vi "AVARVAREI.vi"() -> ()   [LabVIEW 2025]
panel:
  in  "stop":bool
  out "H 4":string
  in  "V 4":bool[](array[boolean])
  out "H2":string
  in  "V 2":bool[](array[boolean])
  out "H 3":string
  in  "V 3":bool[](array[boolean])
  out "H 1":string
  in  "V 1":bool[](array[boolean])
  # "SISTEM DE CONVERSIE DIN BINAR IN HEHAZECIMAL"
  # "CITIREA CODULUI BINAR DE JOS IN SUS/DE LA DREAPTA LA STANGA"
  # "Algoritm de conversie din binar in zecimal\n1 0  0 0 0 1 0 0 (Binar) =132 (Zecimal) = 84 (hexazecimal)\n7 6 5 4 3 2 1 0 - pozitii in sistemul de conversie binar-zecimal\n7 6 5 4 3 2 1 0 - pozitii in vector/ array labVieW\n\n1*2^7+ 0*2^6+.....+ 1*2^2+...0*2^0=132\nMultiply, Add, Power of Two, Subtract\n\nFor loop-parcurgerea elementelor din vector\nN= nr maxim de iteratii=nr elemente vector\n\nIndex Tunnel=inlocuieste utilizarea a 2 functii:\n-index array=permite extragerea elementelor din vector\n-array size\n\nContor i(for loop)=0,1,2,3,4,5,6,7\n\nPower of Two\n-input: contor i\n-output: 2^0, 2^1, 2^2,....\n\nAlgoritm de conversie din zecimal in hexazecimal\n-->apelam functie din LavVIEW - Number to Hexazecimal\n\nShift Registers\n-->acceseaza elementele din iteratiile anterioare(for loop)\n\nBoolean to(0,1)--> conversie T/F la 1/0"
  # "CITIREA CODULUI BINAR DE SUS IN JOS/DE LA STANGA SPRE DREAPTA"
  # "Algoritm de conversie din binar in zecimal\n0 0 1 0 0 0 0 1 (Binar) = 33 (Zecimal) = 21 (hexazecimal)\n7 6 5 4 3 2 1 0 - pozitii in sistemul de conversie binar-zecimal\n0 1 2 3 4 5 6 7- pozitii in vector/ array labVieW\n\nPower of Two\n-input: contor N-1-I\ni=0-->n=8-->n-1-i=8-1-0=7\ni=1-->n=8-->n-1-i=8-1-1=6\n-output: 2^7, 2^6, 2^5....\n\nAlgoritm de conversie din zecimal in hexazecimal\n-->apelam functie din LavVIEW - Number to Hexazecimal"
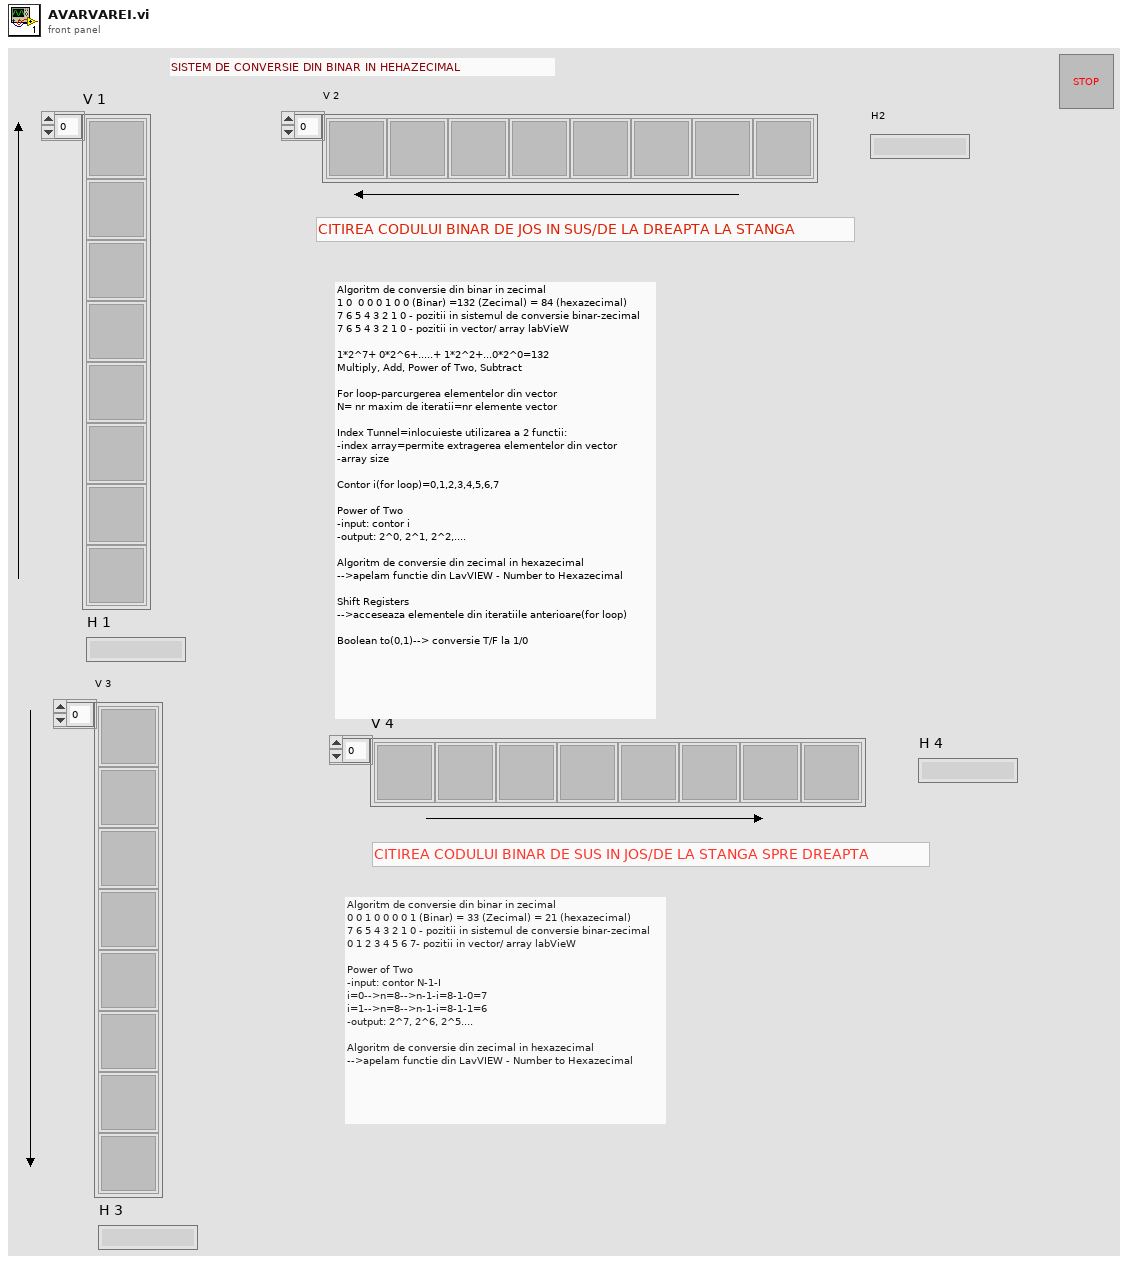
[diagram p1: front panel]
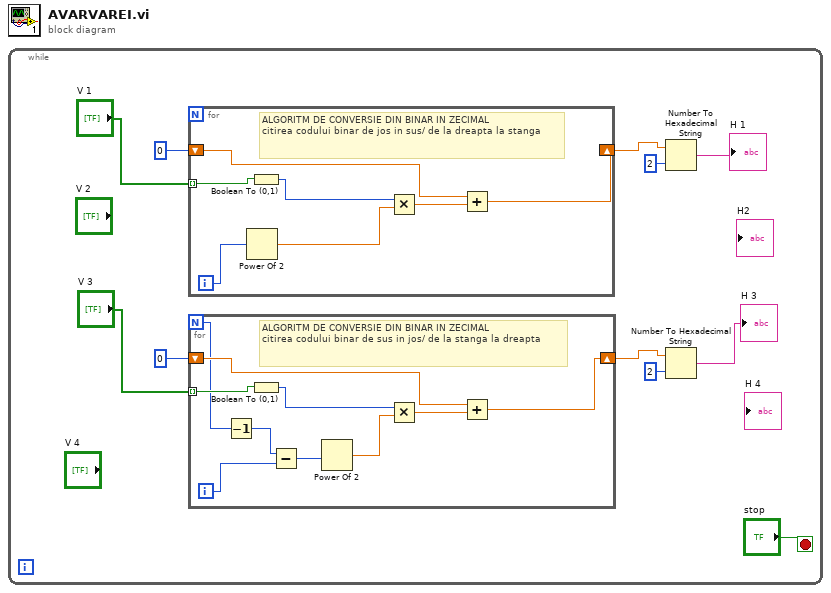
[diagram p0: block diagram]
diagram:
  n1 = while {
    stop <- "stop" stop-if-true
    n2 = for {
      tunnel: "V 1" -> [w28] mode=indexing
      shift-right: [w22] -> w8
      shift-left: 0 -> [w23]
      i -> [w25]
      # "ALGORITM DE CONVERSIE DIN BINAR IN ZECIMAL\ncitirea codului binar de jos in sus/ de la dreapta la stanga"
      n3 = Power Of 2(x=w25) -> (2^x=w26:dbl)
      n4 = Boolean To (0,1)(Boolean=w28) -> (0, 1=w27:i16)
      n5 = Multiply(x=w27, y=w26) -> (x*y=w24:dbl)
      n6 = Add(x=w23, y=w24) -> (x+y=w22:dbl)
    }
    n7 = for {
      N -> [w15]
      tunnel: "V 3" -> [w21] mode=indexing
      shift-right: [w16] -> w4
      shift-left: 0 -> [w17]
      i -> [w13]
      # "ALGORITM DE CONVERSIE DIN BINAR IN ZECIMAL\ncitirea codului binar de sus in jos/ de la stanga la dreapta"
      n8 = Decrement(x=w15) -> (x-1=w14:i32)
      n9 = Boolean To (0,1)(Boolean=w21) -> (0, 1=w20:i16)
      n10 = Subtract(x=w14, y=w13) -> (x-y=w12:i32)
      n11 = Power Of 2(x=w12) -> (2^x=w19:dbl)
      n12 = Multiply(x=w20, y=w19) -> (x*y=w18:dbl)
      n13 = Add(x=w17, y=w18) -> (x+y=w16:dbl)
    }
    n14 = Number To Hexadecimal String(1:i16 2 ("width (-)"), 2:w8) -> (0:→"H 1":string)
    n15 = Number To Hexadecimal String(1:i16 2 ("width (-)"), 2:w4) -> (0:→"H 3":string)
  }
